vi "ConnectReseau.vi"(2 "entrée d'erreur":errorcluster) -> (0 "sortie d'erreur":errorcluster, 1 "Existe?":bool)   [LabVIEW 2015]
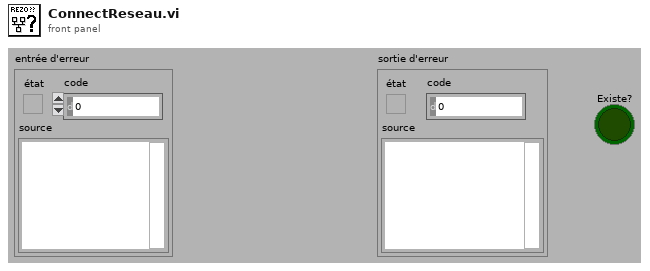
[diagram p1: front panel]
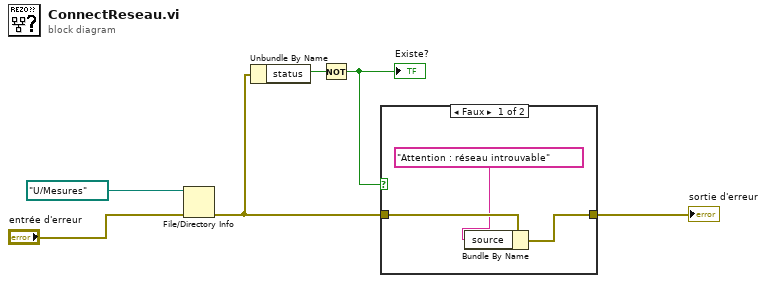
[diagram p0: block diagram]
diagram:
  n1 = File/Directory Info(path=path "U:/Mesures" ("chemin"), error in="entrée d'erreur") -> (error out=w2:errorcluster)  [unwired: 6 out]
  n2 = Unbundle By Name(w2) -> ("status"=w3:bool)
  n3 = Not(x=w3) -> (.not. x?=w5:bool)
  "Existe?" <- w5
  n4 = case shown="Faux" w5 {
    tunnel: w2 -> [w9 w10]
    tunnel: [w7 w10] -> w1
    frame False {
      n5 = Bundle By Name(cluster=w9, "source"="Attention : réseau introuvable") -> (w7:errorcluster)
    }
    frame True {
    }
  }
  "sortie d'erreur" <- w1
